vi "RNN_full_iteration.vi"() -> ()   [LabVIEW 2014]
uses:
  <vilib>/Analysis/Matrix/Datatypes/RealMatrix.ctl
  <vilib>/Analysis/Matrix/Numeric/Conversions/Matrix To Array - RM.vi
  <vilib>/Analysis/Matrix/Numeric/Conversions/Array To Matrix - RA2.vi
  <vilib>/Analysis/Matrix/NI_Matrix.lvlib
panel:
  out "params_":T2
  in  "learning_rate":dbl
  out "dParams_":T3
  in  "targets":i64[](array[numeric])=[0]
  in  "_inputs":i32[](array[numeric])
  in  "_params":T2
  in  "_hprev":T1
  in  "_vocab size":i32
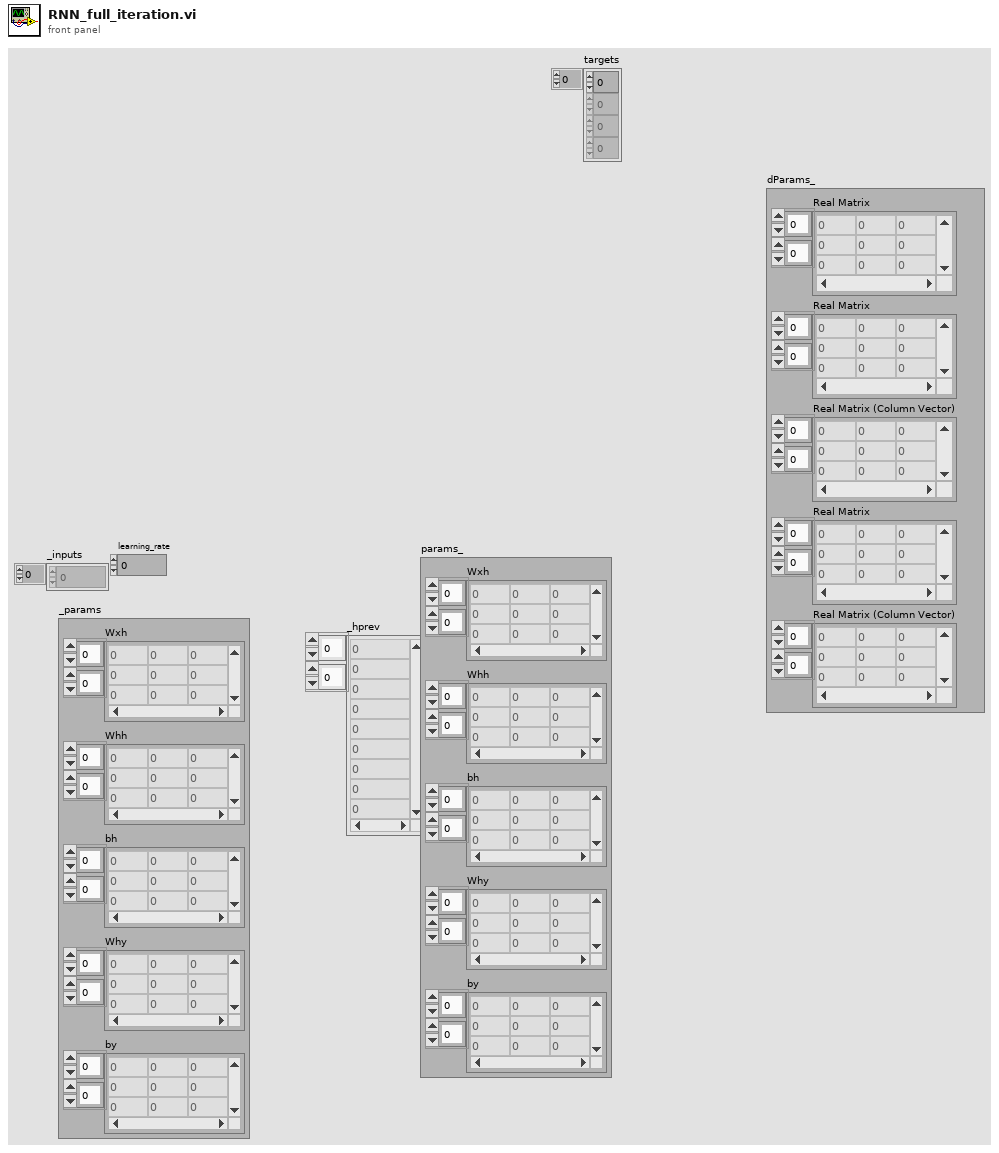
[diagram p1: front panel]
types:
  T1 = typedef "NI_Matrix.lvlib/RealMatrix.ctl" = dbl[][]
  T2 = cluster{"Wxh":T1, "Whh":T1, "bh":T1, "Why":T1, "by":T1}
  T3 = cluster{"Real Matrix":T1, "Real Matrix":T1, "Real Matrix (Column Vector)":T1, "Real Matrix":T1, "Real Matrix (Column Vector)":T1}
  T4 = cluster{"dWxh":T1, "dWhh":T1, "dbh":T1, "dWhy":T1, "dby":T1}
  T5 = cluster{"Real Matrix":T1, "Real Matrix":T1, "Real Matrix":T1, "Real Matrix":T1, "Real Matrix":T1}
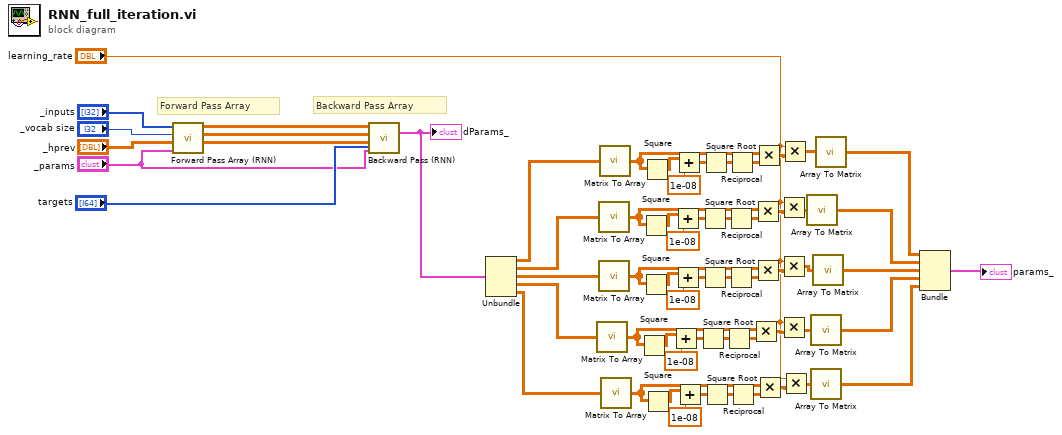
[diagram p0: block diagram]
diagram:
  # "Backward Pass Array"
  # "Forward Pass Array"
  n1 = call "Forward Pass Array (RNN).vi"("inputs"="_inputs", "vocab size"="_vocab size", "hprev"="_hprev", "params_"="_params") -> ("xs"=w57:dbl[][][], "hs"=w56:dbl[][][], "ps"=w55:dbl[][][])  [unwired: 3 in, 1 out]
  n2 = call "Backward Pass (RNN).vi"("xs"=w57, "hs"=w56, "ps"=w55, "targets"="targets", "params"="_params") -> ("dParams_"=w53:T4)  [unwired: 10 in]
  "dParams_" <- w53
  n3 = Unbundle(w53) -> ("dWxh"=w52:T1, "dWhh"=w16:T1, "dbh"=w15:T1, "dWhy"=w14:T1, "dby"=w13:T1)
  n4 = call-poly <vilib>:"Matrix To Array.vi"("Real Matrix"=w14) -> ("Real 2D Array"=w28:dbl[][])
  n5 = call-poly <vilib>:"Matrix To Array.vi"("Real Matrix"=w16) -> ("Real 2D Array"=w42:dbl[][])
  n6 = call-poly <vilib>:"Matrix To Array.vi"("Real Matrix"=w15) -> ("Real 2D Array"=w35:dbl[][])
  n7 = call-poly <vilib>:"Matrix To Array.vi"("Real Matrix"=w52) -> ("Real 2D Array"=w49:dbl[][])
  n8 = call-poly <vilib>:"Matrix To Array.vi"("Real Matrix"=w13) -> ("Real 2D Array"=w21:dbl[][])
  n9 = Square(x=w28) -> (x^2=w24:dbl[][])
  n10 = Square(x=w42) -> (x^2=w38:dbl[][])
  n11 = Square(x=w35) -> (x^2=w31:dbl[][])
  n12 = Square(x=w49) -> (x^2=w45:dbl[][])
  n13 = Square(x=w21) -> (x^2=w17:dbl[][])
  n14 = Add(x=w24, y=1e-08 ("x")) -> (x+y=w30:dbl[][])
  n15 = Add(x=w38, y=1e-08 ("x")) -> (x+y=w44:dbl[][])
  n16 = Add(x=w31, y=1e-08 ("x")) -> (x+y=w37:dbl[][])
  n17 = Add(x=w45, y=1e-08 ("x")) -> (x+y=w51:dbl[][])
  n18 = Add(x=w17, y=1e-08 ("x")) -> (x+y=w23:dbl[][])
  n19 = Square Root(x=w30) -> (sqrt(x)=w29:dbl[][])
  n20 = Square Root(x=w44) -> (sqrt(x)=w43:dbl[][])
  n21 = Square Root(x=w37) -> (sqrt(x)=w36:dbl[][])
  n22 = Square Root(x=w51) -> (sqrt(x)=w50:dbl[][])
  n23 = Square Root(x=w23) -> (sqrt(x)=w22:dbl[][])
  n24 = Reciprocal(x=w29) -> (1/x=w27:dbl[][])
  n25 = Reciprocal(x=w43) -> (1/x=w41:dbl[][])
  n26 = Reciprocal(x=w36) -> (1/x=w34:dbl[][])
  n27 = Reciprocal(x=w50) -> (1/x=w48:dbl[][])
  n28 = Reciprocal(x=w22) -> (1/x=w20:dbl[][])
  n29 = Multiply(x=w28, y=w27) -> (x*y=w26:dbl[][])
  n30 = Multiply(x=w42, y=w41) -> (x*y=w40:dbl[][])
  n31 = Multiply(x=w35, y=w34) -> (x*y=w33:dbl[][])
  n32 = Multiply(x=w49, y=w48) -> (x*y=w47:dbl[][])
  n33 = Multiply(x=w21, y=w20) -> (x*y=w19:dbl[][])
  n34 = Multiply(x="learning_rate", y=w40) -> (x*y=w7:dbl[][])
  n35 = Multiply(x="learning_rate", y=w33) -> (x*y=w8:dbl[][])
  n36 = Multiply(x="learning_rate", y=w26) -> (x*y=w9:dbl[][])
  n37 = Multiply(x="learning_rate", y=w47) -> (x*y=w11:dbl[][])
  n38 = Multiply(x="learning_rate", y=w19) -> (x*y=w10:dbl[][])
  n39 = call-poly <vilib>:"Array To Matrix.vi"("Real 2D Array"=w7) -> ("Real Matrix"=w5:T1)
  n40 = call-poly <vilib>:"Array To Matrix.vi"("Real 2D Array"=w9) -> ("Real Matrix"=w3:T1)
  n41 = call-poly <vilib>:"Array To Matrix.vi"("Real 2D Array"=w10) -> ("Real Matrix"=w2:T1)
  n42 = call-poly <vilib>:"Array To Matrix.vi"("Real 2D Array"=w8) -> ("Real Matrix"=w4:T1)
  n43 = call-poly <vilib>:"Array To Matrix.vi"("Real 2D Array"=w11) -> ("Real Matrix"=w6:T1)
  n44 = Bundle("Real Matrix"=w6, "Real Matrix"=w5, "Real Matrix"=w4, "Real Matrix"=w3, "Real Matrix"=w2) -> (→"params_":T5)  [unwired: 1 in]
